vi "Compute Chirp Parameters.vi"(8 "Error in":errorcluster) -> (0 "error out":errorcluster, 3 "Chirp parameters (all Z planes)":cluster{"HexPackets":string[]}[](array[cluster]))   [LabVIEW 2020]
uses:
  Typedefs/Controls/AOL_Globals.ctl
  Typedefs/Imaging Protocols enum.ctl
  Typedefs/Frame Size.ctl
  Typedefs/AOL modes.ctl
  Typedefs/Plane Mode.ctl
  Typedefs/Functional Mode.ctl
  Global Variables/General Globals.vi
panel:
  out "AOL_Globals":T1={"Imaging Protocol"=enum."Live Imaging", "Number of POI"=0, "Number of Miniscans"=0, "Number of Trials"=0, "Number of Cycles "=0, "# Averaged Frames"=0, "Laser power (%)"=0, "Pockels (V)"=0.0, "Acquisition Length (sec)"=0.0, "Fill time (us)"=0.0, "POI Dwell time (us)"=0.0, "Miniscan Dwell time per pixel (us)"=0.0, "PMT 1"=0.0, "PMT 2"=0.0, "Back Apperture (mA)"=0.0, "Frame Size"=200, "Center Frequency"=0.0, "Field of View (um)"=175.0, "Field of View (norm)"=0.0, "DwellTime (us)"=0.0, "Ref Dwell Time (us)"=0.0, "Wavelength (nm)"=0.0, "Zoom"=0.0, "AOL Z"=0.0, "AOL Mode"=enum."Raster", "GridXY"=0.0, "GridZ"=0.0, "TriggerPeriod (sec)"=0.0, "Number of Pixels in Miniscan"=0, "Experiment folder path"=path "", "X centre"=0.0, "Y centre"=0.0, "Angle (degrees)"=0.0, "Angle Xs (degrees)"=0.0, "Angle Ys (degrees)"=0.0, "Plane Mode"=0, "Threshold"=[], "Regenerate Chirps"=FALSE, "Rectangle ROI length (pixels)"=0, "Rectangle ROI height (pixels)"=0, "AOD fill"=4900, "StartupDelay"=0, "Samples Wait after Trigger"=5080, "Slip Cycle"=600000, "Add Cycle"=TRUE, "Functional Mode"=enum."Point", "Z Start"=0.0, "Z Stop"=0.0, "# Planes"=0, "Total Pixels"=0, "Variable Miniscan Pixels"=[], "Use Variable Length"=FALSE, "Use Variable Resolution"=FALSE, "Laser power (%) at Z Start"=0, "Laser power (%) at Z Stop"=0, "Ref Z Step"=0} {"Angle Ys (degrees)" format="%#.6g"; "Angle Xs (degrees)" format="%#.6g"; "Plane Mode" items=["XY Plane", "XZ Plane", "YZ Plane", "arbitraryplane"]; "Frame Size" items=["100X100"=100, "128X128"=128, "200X200"=200, "256X256"=256, "512X512"=512, "1024x1024"=1024, "2048x2048"=2048]; "Back Apperture (mA)" format="%#.6g"; "Pockels (V)" format="%#.6g"; "PMT 2" format="%#.6g"; "PMT 1" format="%#.6g"; "Angle (degrees)" format="%#.6g"; "POI Dwell time (us)" format="%#.6g"}
  out "Values change check loop":i32
  out "Generator loop":i32
  out "Regenerating Chirps":bool
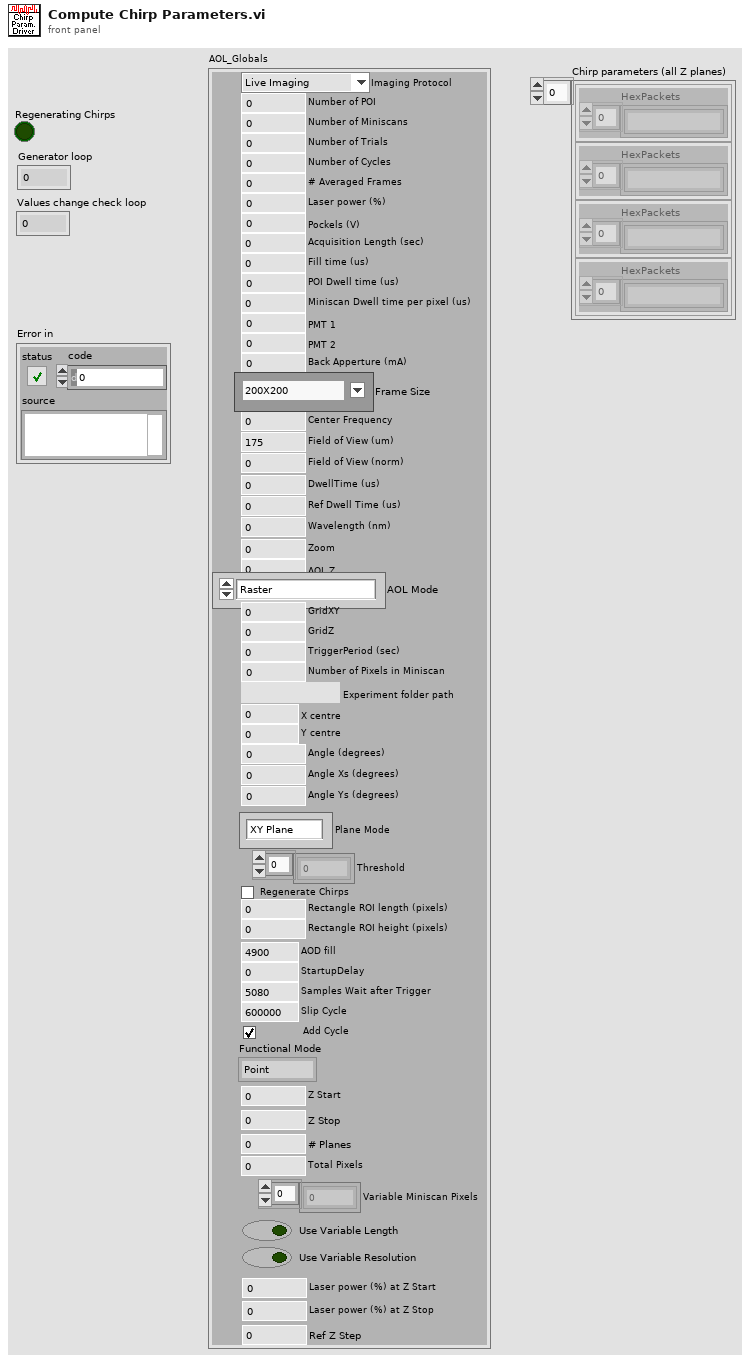
[diagram p1: front panel]
types:
  T1 = typedef "AOL_Globals.ctl" = cluster{"Imaging Protocol":T2, "Number of POI":u16, "Number of Miniscans":u16, "Number of Trials":u16, "Number of Cycles ":u64, "# Averaged Frames":u16, "Laser power (%)":u8, "Pockels (V)":dbl, "Acquisition Length (sec)":dbl, "Fill time (us)":dbl, "POI Dwell time (us)":dbl, "Miniscan Dwell time per pixel (us)":dbl, "PMT 1":dbl, "PMT 2":dbl, "Back Apperture (mA)":dbl, "Frame Size":T3, "Center Frequency":dbl, "Field of View (um)":dbl, "Field of View (norm)":dbl, "DwellTime (us)":dbl, "Ref Dwell Time (us)":dbl, "Wavelength (nm)":dbl, "Zoom":dbl, "AOL Z":dbl, "AOL Mode":T4, "GridXY":dbl, "GridZ":dbl, "TriggerPeriod (sec)":dbl, "Number of Pixels in Miniscan":u16, "Experiment folder path":path, "X centre":dbl, "Y centre":dbl, "Angle (degrees)":dbl, "Angle Xs (degrees)":dbl, "Angle Ys (degrees)":dbl, "Plane Mode":T5, "Threshold":u16[], "Regenerate Chirps":bool, "Rectangle ROI length (pixels)":u16, "Rectangle ROI height (pixels)":u16, "AOD fill":u16, "StartupDelay":i32, "Samples Wait after Trigger":u16, "Slip Cycle":u32, "Add Cycle":bool, "Functional Mode":T6, "Z Start":dbl, "Z Stop":dbl, "# Planes":i32, "Total Pixels":i32, "Variable Miniscan Pixels":u16[], "Use Variable Length":bool, "Use Variable Resolution":bool, "Laser power (%) at Z Start":u8, "Laser power (%) at Z Stop":u8, "Ref Z Step":i8}
  T2 = typedef "Imaging Protocols enum.ctl" = enum16{"AOL Z-Stack", "Motor Z Stack", "Parameter Sweep", "Functional Acquisition", "Single Plane Acquisition", "Volume Acquisition", "Live Imaging", "Live Plane Imaging", "Live Volume Imaging"}
  T3 = typedef "Frame Size.ctl" = u16
  T4 = typedef "AOL modes.ctl" = enum16{"Raster", "Structural", "Pointing", "Mini Scan", "Alignment"}
  T5 = typedef "Plane Mode.ctl" = u16
  T6 = typedef "Functional Mode.ctl" = enum16{"Point", "Line", "Patch", "Plane", "Volume"}
  T7 = cluster{"ZStack":cluster{"Zstart":dbl, "Zstop":dbl, "Zstep":dbl}, "Laser Power %":cluster{"@ Start":dbl, "@ Stop":dbl}}
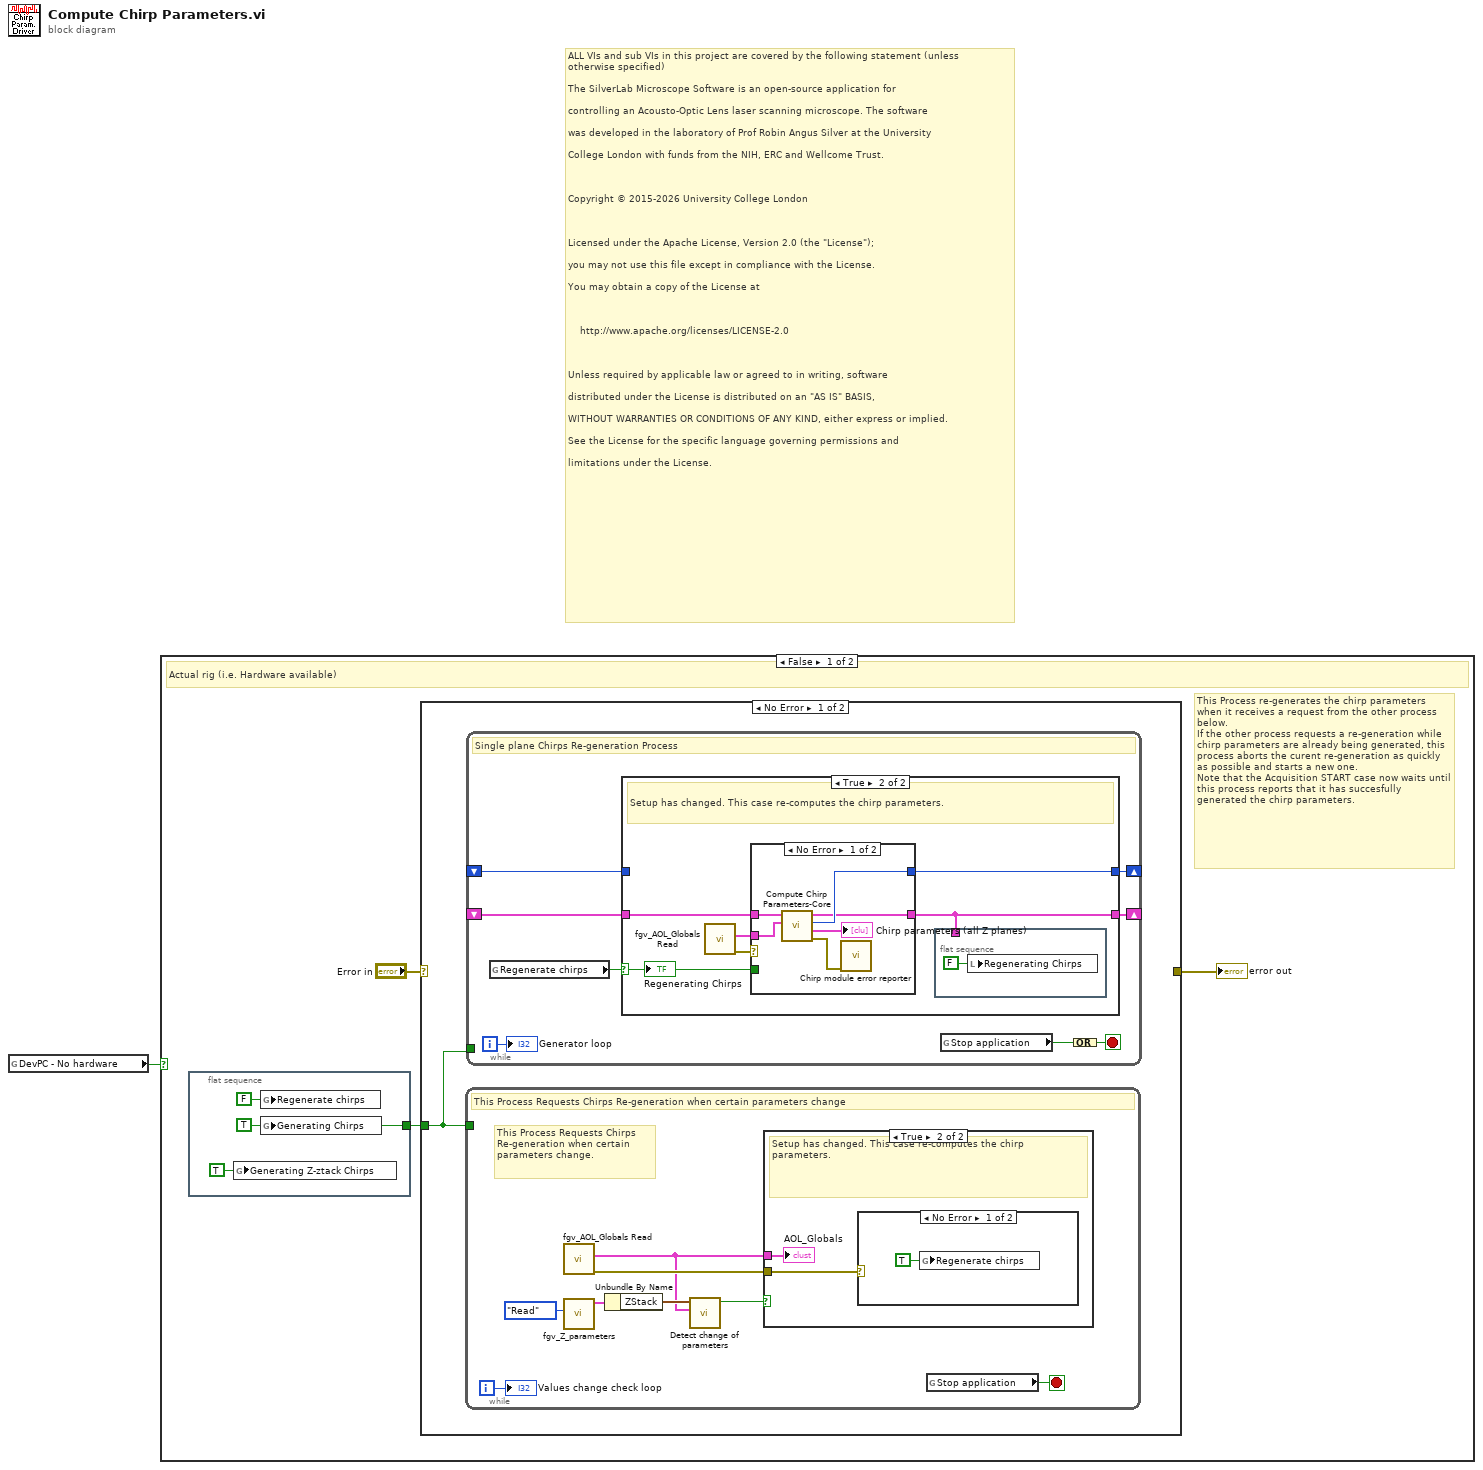
[diagram p0: block diagram]
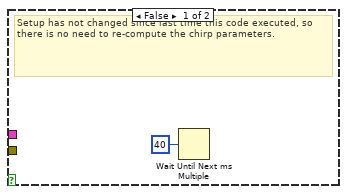
[diagram p2: hidden frame]
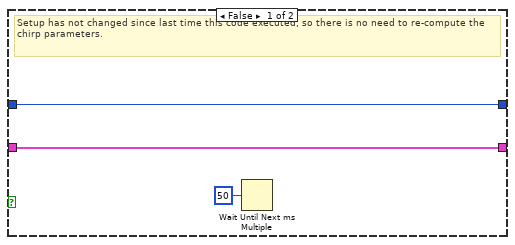
[diagram p4: hidden frame]
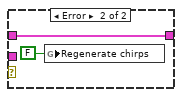
[diagram p5: hidden frame]
diagram:
  # "ALL VIs and sub VIs in this project are covered by the following statement (unless \notherwise specified)\n\nThe SilverLab Microscope Software is an open-source application for\n\ncontrolling an Acousto-Optic Lens laser scanning microscope. The software\n\nwas developed in the laboratory of Prof Robin Angus Silver at the University\n\nCollege London with funds from the NIH, ERC and Wellcome Trust.\n\n \n\nCopyright © 2015-2026 University College London\n\n \n\nLicensed under the Apache License, Version 2.0 (the \"License\");\n\nyou may not use this file except in compliance with the License.\n\nYou may obtain a copy of the License at\n\n \n\n    http://www.apache.org/licenses/LICENSE-2.0\n\n \n\nUnless required by applicable law or agreed to in writing, software\n\ndistributed under the License is distributed on an \"AS IS\" BASIS,\n\nWITHOUT WARRANTIES OR CONDITIONS OF ANY KIND, either express or implied.\n\nSee the License for the specific language governing permissions and\n\nlimitations under the License."
  n1 = global read "General Globals.vi" "DevPC - No hardware"() -> (w1:bool)
  n2 = case shown="False" w1 {
    frame False {
      # "This Process re-generates the chirp parameters when it receives a request from the other process below.\nIf the other process requests a re-generation while chirp parameters are already being generated, this process aborts the curent re-generation as quickly as possible and starts a new one.\nNote that the Acquisition START case now waits until this process reports that it has succesfully generated the chirp parameters."
      # "Actual rig (i.e. Hardware available)"
      n3 = flat-sequence {
        tunnel: [w47] -> w2
        frame #0 {
          w47 = TRUE ("Generating Chirps")
          n4 = global write "General Globals.vi" "Generating Z-ztack Chirps"(TRUE ("Generating Chirps")) -> ()
          n5 = global write "General Globals.vi" "Regenerate chirps"(FALSE ("Regenerate chirps")) -> ()
          n6 = global write "General Globals.vi" "Generating Chirps"(w47) -> ()
        }
      }
      n7 = case shown="No Error" "Error in" {
        selector: "Error in" -> [_ w44]
        tunnel: w2 -> [w5 _]
        tunnel: [_ w44] -> w4
        frame No Error {
          n8 = while {
            tunnel: w5 -> [_]
            i -> [w7]
            stop <- w8 stop-if-true
            # "This Process Requests Chirps Re-generation when certain parameters change."
            # "This Process Requests Chirps Re-generation when certain parameters change"
            n9 = call "fgv_AOL_Globals Read.vi"() -> ("error out"=w13:errorcluster, "AOL_Globals"=w6:T1)  [unwired: 9 in, 1 out]
            n10 = call "fgv_Z_parameters.vi"("Function"=enum16{"Intialize", "Write", "Read", "Clear"}."Read") -> ("Z Parameters"=w11:T7)  [unwired: 9 in, 1 out]
            n11 = Unbundle By Name(w11) -> ("ZStack"=w10:cluster{"Zstart":dbl, "Zstop":dbl, "Zstep":dbl})
            n12 = call "Detect change of parameters.vi"("AOL_Globals"=w6, "ZStack"=w10) -> ("Setup has changed"=w9:bool)  [unwired: 9 in]
            n13 = case shown="True" w9 {
              tunnel: w13 -> [_ w16]
              tunnel: w6 -> [_ w15]
              frame False {
                # "Setup has not changed since last time this code executed, so there is no need to re-compute the chirp parameters."
                n14 = Wait Until Next ms Multiple(millisecond multiple=u32 40) -> ()  [unwired: 1 out]
              }
              frame True {
                # "Setup has changed. This case re-computes the chirp parameters."
                n15 = case shown="No Error" w16 {
                  frame No Error {
                    n16 = global write "General Globals.vi" "Regenerate chirps"(TRUE ("Regenerate chirps")) -> ()
                  }
                  frame Error {
                  }
                }
                "AOL_Globals" <- w15
              }
            }
            n17 = global read "General Globals.vi" "Stop application"() -> (w8:bool)
            "Values change check loop" <- w7
          }
          n18 = while {
            shift-right: [w25] -> _
            shift-left: _ -> [w24]
            tunnel: w5 -> [_]
            shift-right: [w21] -> _
            shift-left: _ -> [w20]
            i -> [w22]
            stop <- w18 stop-if-true
            # "Single plane Chirps Re-generation Process"
            n19 = global read "General Globals.vi" "Regenerate chirps"() -> (w23:bool)
            n20 = case shown="True" w23 {
              selector: w23 -> [_ w31]
              tunnel: [w28 w34] -> w25
              tunnel: w24 -> [w28 _]
              tunnel: [w26 w29] -> w21
              tunnel: w20 -> [w26 w30]
              frame False {
                # "Setup has not changed since last time this code executed, so there is no need to re-compute the chirp parameters."
                n21 = Wait Until Next ms Multiple(millisecond multiple=u32 50) -> ()  [unwired: 1 out]
              }
              frame True {
                # "Setup has changed. This case re-computes the chirp parameters."
                n22 = call "fgv_AOL_Globals Read.vi"() -> ("error out"=w32:errorcluster, "AOL_Globals"=w33:T1)  [unwired: 9 in, 1 out]
                n23 = case shown="No Error" w32 {
                  tunnel: [w41 _] -> w34
                  tunnel: w33 -> [w37 _]
                  tunnel: w31 -> [_ _]
                  tunnel: [w40 w42] -> w29
                  tunnel: w30 -> [w39 w42]
                  frame No Error {
                    n24 = call "Compute Chirp Parameters-Core.vi"("AOL_Globals"=w37, "Chirp in"=w39) -> ("error out"=w36:errorcluster, "Z-stack chirp parameters"=→"Chirp parameters (all Z planes)":cluster{"HexPackets":string[]}[], "# of Z-planes"=w41:i32, "Chirp out"=w40:cluster{"HexPackets":string[]})  [unwired: 6 in]
                    n25 = call "Chirp module error reporter.vi"("error in (no error)"=w36) -> ()  [unwired: 11 in]
                  }
                  frame Error {
                    n26 = global write "General Globals.vi" "Regenerate chirps"(FALSE ("Regenerate chirps")) -> ()
                  }
                }
                n27 = flat-sequence {
                  tunnel: w29 -> [_]
                  frame #0 {
                    n28 = local write "Regenerating Chirps"(FALSE ("Regenerating Chirps")) -> ()
                  }
                }
                "Regenerating Chirps" <- w31
              }
            }
            n29 = global read "General Globals.vi" "Stop application"() -> (w19:bool)
            n30 = Compound Arithmetic op=OR(w19) -> (w18:bool)
            "Generator loop" <- w22
          }
        }
        frame Error {
        }
      }
      "error out" <- w4
    }
    frame True {
      # "Development Computer (i.e. No hardware available)"
    }
  }
